vi "TestReport_getData.vi"(0 "ReportPath":path) -> (1 "TableData":T2[](array[typedef]), 2 "ImageData":T1[](array[typedef]))   [LabVIEW 2016]
uses:
  WorReport_tableData.ctl
  WorReport_imageData.ctl
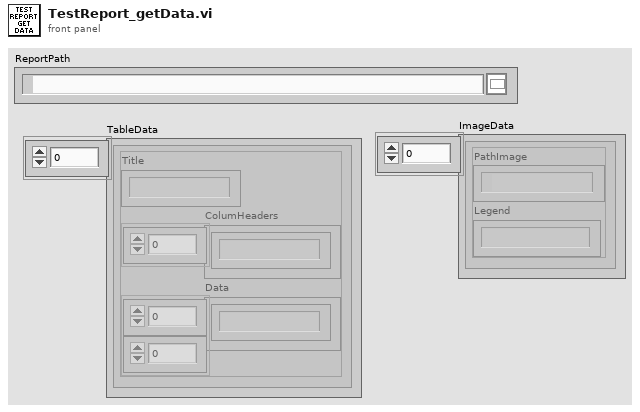
[diagram p1: front panel]
types:
  T1 = typedef "WorReport_imageData.ctl" = cluster{"PathImage":path, "Legend":string}
  T2 = typedef "WorReport_tableData.ctl" = cluster{"Title":string, "ColumHeaders":string[], "Data":string[][]}
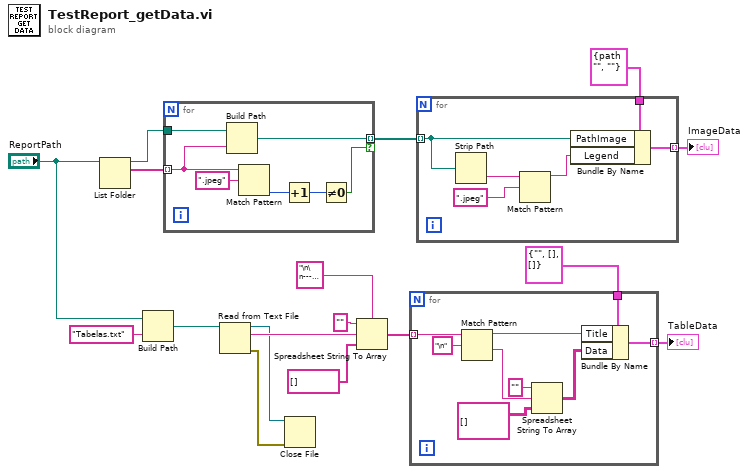
[diagram p0: block diagram]
diagram:
  n1 = List Folder(path="ReportPath") -> (path out=w16:path, filenames=w17:string[])  [unwired: 3 in, 2 out]
  n2 = Build Path(base path="ReportPath", name or relative path="Tabelas.txt") -> (appended path=w11:path)
  n3 = for {
    tunnel: w17 -> [w21] mode=indexing
    tunnel: w16 -> [w20]
    tunnel: [w19] -> w15 mode=indexing if=w18
    n4 = Build Path(base path=w20, name or relative path=w21) -> (appended path=w19:path)
    n5 = Match Pattern(string=w21, regular expression=".jpeg") -> (offset past match=w23:i32)  [unwired: 1 in, 3 out]
    n6 = Increment(x=w23) -> (x+1=w22:i32)
    n7 = Not Equal To 0?(x=w22) -> (x != 0?=w18:bool)
  }
  n8 = Read from Text File(file (use dialog)=w11) -> (refnum out=w6:refnum<file>, text=w7:string, error out=w5:errorcluster)  [unwired: 3 in, 1 out]
  n9 = Close File(refnum=w6, error in=w5) -> ()  [unwired: 2 out]
  n10 = Spreadsheet String To Array(delimiter (Tab)="\n\n---   ---   ---   ---   ---   ---   ---   ---   ---   ---   \n\n" ("string"), format string="", spreadsheet string=w7, array type (2D Dbl)=string[] [] ("format string")) -> (array=w4:string[])
  n11 = for {
    tunnel: w4 -> [w32] mode=indexing
    tunnel: T2 {"Title"="", "ColumHeaders"=[], "Data"=[]} ("tableData") -> [w31]
    tunnel: [w25] -> w2 mode=indexing
    n12 = Match Pattern(string=w32, regular expression="\n") -> (before substring=w30:string, after substring=w29:string)  [unwired: 1 in, 2 out]
    n13 = Spreadsheet String To Array(format string="", spreadsheet string=w29, array type (2D Dbl)=string[][] [] ("format string")) -> (array=w26:string[][])  [unwired: 1 in]
    n14 = Bundle By Name(cluster=w31, "Title"=w30, "Data"=w26) -> (w25:T2)
  }
  "TableData" <- w2
  n15 = for {
    tunnel: w15 -> [w38] mode=indexing
    tunnel: T1 {"PathImage"=path "", "Legend"=""} ("imageData") -> [w39]
    tunnel: [w34] -> w1 mode=indexing
    n16 = Strip Path(path=w38) -> (name=w36:string)  [unwired: 1 out]
    n17 = Match Pattern(string=w36, regular expression=".jpeg") -> (before substring=w35:string)  [unwired: 1 in, 3 out]
    n18 = Bundle By Name(cluster=w39, "PathImage"=w38, "Legend"=w35) -> (w34:T1)
  }
  "ImageData" <- w1
